vi "Reset.vi"(8 "error in (no error)":errorcluster, 11 "Settle Output in":refnum<class "Settle Output.lvclass">) -> (0 "error out":errorcluster, 3 "Settle Output out":refnum<class "Settle Output.lvclass">)   [LabVIEW 2015, in "Settle Output.lvclass"]
uses:
  Settle Output.lvclass
  Settle Output.lvclass/Settle Output.ctl
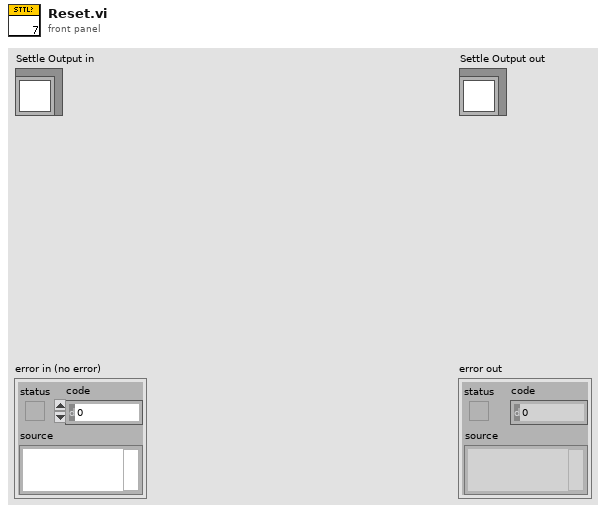
[diagram p1: front panel]
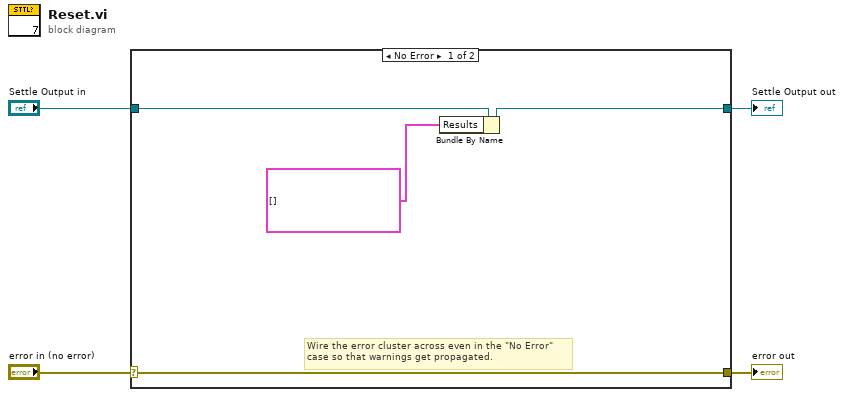
[diagram p0: block diagram]
diagram:
  n1 = case shown="No Error" "error in (no error)" {
    selector: "error in (no error)" -> [w7 w10]
    tunnel: [w7 w10] -> w3
    tunnel: [w6 w9] -> w1
    tunnel: "Settle Output in" -> [w8 w9]
    frame No Error {
      # "Wire the error cluster across even in the \"No Error\"\ncase so that warnings get propagated."
      n2 = Bundle By Name(cluster=w8, "Results"=cluster{"Time Stamp":timestamp, "Result":dbl}[] []) -> (w6:refnum<class "Settle Output.lvclass">)
    }
    frame Error {
    }
  }
  "error out" <- w3
  "Settle Output out" <- w1
